vi "Read Name.vi"(11 "Log Sinks in":refnum<class "Log Sinks.lvclass">) -> (2 "Name":string, 3 "Log Sinks out":refnum<class "Log Sinks.lvclass">)   [LabVIEW 2019, in "TSC Event Logger.lvlib" / "Log Sinks.lvclass"]
doc: "Data Member Access method to read the name of the sink.\n\n<b>Code Developed By:</b>\nTechnology Service Corporation\nBloomington, IN 47403\nwww.tsc.com/atcs\n\nDeveloper:\nDaniel Coons"
uses:
  Log Sinks.lvclass
  Log Sinks.lvclass/Log Sinks.ctl
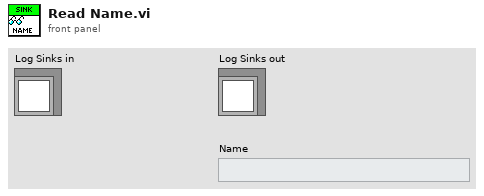
[diagram p1: front panel]
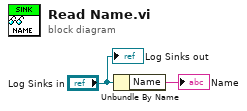
[diagram p0: block diagram]
diagram:
  n1 = Unbundle By Name("Log Sinks in") -> ("Name"=→"Name":string)
  "Log Sinks out" <- "Log Sinks in"
